vi "Identificar_todos_los_switches.vi"(11 "Response 8bit":string) -> (2 "number":u32, 3 "Array":bool[](array[boolean]))   [LabVIEW 2019]
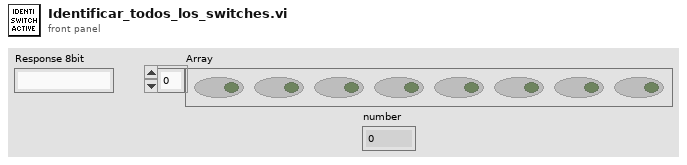
[diagram p1: front panel]
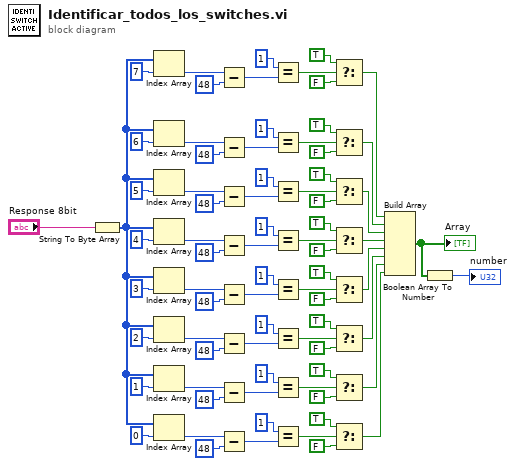
[diagram p0: block diagram]
diagram:
  n1 = String To Byte Array(string="Response 8bit") -> (unsigned byte array=w68:u8[])
  n2 = Index Array(array=w68, index=7) -> (element=w43:u8)
  n3 = Index Array(array=w68, index=6) -> (element=w45:u8)
  n4 = Index Array(array=w68, index=5) -> (element=w47:u8)
  n5 = Index Array(array=w68, index=4) -> (element=w49:u8)
  n6 = Index Array(array=w68, index=3) -> (element=w51:u8)
  n7 = Index Array(array=w68, index=2) -> (element=w53:u8)
  n8 = Index Array(array=w68, index=1) -> (element=w55:u8)
  n9 = Index Array(array=w68, index=0) -> (element=w58:u8)
  n10 = Subtract(x=w43, y=u8 48) -> (x-y=w8:u8)
  n11 = Subtract(x=w45, y=u8 48) -> (x-y=w13:u8)
  n12 = Subtract(x=w47, y=u8 48) -> (x-y=w18:u8)
  n13 = Subtract(x=w49, y=u8 48) -> (x-y=w23:u8)
  n14 = Subtract(x=w51, y=u8 48) -> (x-y=w28:u8)
  n15 = Subtract(x=w53, y=u8 48) -> (x-y=w33:u8)
  n16 = Subtract(x=w55, y=u8 48) -> (x-y=w42:u8)
  n17 = Subtract(x=w58, y=u8 48) -> (x-y=w3:u8)
  n18 = Equal?(x=u8 1, y=w8) -> (x = y?=w11:bool)
  n19 = Equal?(x=u8 1, y=w13) -> (x = y?=w16:bool)
  n20 = Equal?(x=u8 1, y=w18) -> (x = y?=w21:bool)
  n21 = Equal?(x=u8 1, y=w23) -> (x = y?=w26:bool)
  n22 = Equal?(x=u8 1, y=w28) -> (x = y?=w31:bool)
  n23 = Equal?(x=u8 1, y=w33) -> (x = y?=w36:bool)
  n24 = Equal?(x=u8 1, y=w42) -> (x = y?=w40:bool)
  n25 = Equal?(x=u8 1, y=w3) -> (x = y?=w6:bool)
  n26 = Select(t=TRUE, s=w11, f=FALSE) -> (s? t:f=w76:bool)
  n27 = Select(t=TRUE, s=w16, f=FALSE) -> (s? t:f=w75:bool)
  n28 = Select(t=TRUE, s=w21, f=FALSE) -> (s? t:f=w74:bool)
  n29 = Select(t=TRUE, s=w26, f=FALSE) -> (s? t:f=w73:bool)
  n30 = Select(t=TRUE, s=w31, f=FALSE) -> (s? t:f=w72:bool)
  n31 = Select(t=TRUE, s=w36, f=FALSE) -> (s? t:f=w71:bool)
  n32 = Select(t=TRUE, s=w40, f=FALSE) -> (s? t:f=w70:bool)
  n33 = Select(t=TRUE, s=w6, f=FALSE) -> (s? t:f=w69:bool)
  n34 = Build Array(w76, w75, w74, w73, w72, w71, w70, w69) -> (w2:bool[])
  "Array" <- w2
  n35 = Boolean Array To Number(Boolean array=w2) -> (number=→"number":u32)
